vi "Npsv pc test.vi"() -> ()   [LabVIEW 2019]
uses:
  Reverse Polarity.ctl
  Forward Polarity.ctl
  Motion Controller Slot.ctl
  Stepper Output Configuration.ctl
  Axis Select.ctl
  MsgTypeDef.ctl
  DataDef.ctl
  <vilib>/NI/Modbus Library/API/Modbus API.lvclass
  <vilib>/WPC Systems Ltd/GECO Driver/Lib/GECOBase/GECO_Driver Class/GECO_Driver.lvclass
  <vilib>/WPC Systems Ltd/GECO Driver/Lib/GECOMotion/GECOMotion/_typedefine/Axis Select.ctl
  <vilib>/WPC Systems Ltd/GECO Driver/Lib/GECOBase/GECO_Driver Class/Motion/_typedefine/GECO_Stepper Output Configuration.ctl
  <vilib>/WPC Systems Ltd/GECO Driver/Lib/GECOBase/GECO_Driver Class/Motion/_typedefine/GECO_Motion Operation Mode.ctl
  <vilib>/WPC Systems Ltd/GECO Driver/Lib/GECOBase/GECO_Driver Class/GECO_SlotName.ctl
  <vilib>/WPC Systems Ltd/GECO Driver/Lib/GECOBase/GECO_Driver Class/Motion/_typedefine/GECO_ActiveHighLow.ctl
  <vilib>/WPC Systems Ltd/GECO Driver/Lib/GECOMotion/GECOMotion/GECO Motion.lvclass
  GyroDef.ctl
  <vilib>/Instr/_visa.llb/VISA Configure Serial Port (Instr).vi
panel:
  out "RT error out":errorcluster
  out "RT Program Period":u32
  out "error IO 2":errorcluster
  out "error IO":errorcluster
  out "實際角度":cluster{"A":dbl, "B":dbl}={"A"=-3.299667554384925, "B"=3.520332445615068}
  out "實際角度Chart":cluster{"X":dbl, "Y":dbl}(graph)={"X"=-3.299667554384925, "Y"=3.520332445615068} caption="Waveform Chart - dark"
  out "Gyro\nPeriod":u32
  in  "Main Setting Tab":T1(tab)
  in  "TimerON":bool
  in  "Timer(ms)":i32=1
  in  "Serial Port":refnum<visa-resource-name>="COM3"
  in  "TCP slave port":u32=1
  in  "baud rate":u32=115200
  in  "Byte bits":u32=8
  in  "Modbus Address Starting":u32
  in  "Modbus Number of Inputs":u32=10000
  in  "Resource Name":tag="rio://192.168.0.224/RIO0"
  in  "Servo on":bool
  in  "Axis Select":T2
  in  "Stepper Output Configuration":T3=enum."CW/CCW(Two Pulse)"
  in  "Forward Enable?":bool=TRUE
  in  "Reverse Enable?":bool=TRUE
  in  "Motion Operation Mode":T4(ring)=enum."Velocity"
  in  "Forward Polarity":T5
  in  "Reverse Polarity":T6
  in  "Motion Controller Slot":T7
  in  "Target Position (0)":dbl=10000.0
  in  "Acceleration (100000)":u32=300000
  in  "Velocity (10000)":dbl=100000.0
  in  "Deacceleration (100000)":u32=300000
  in  "PID gains setting Tab":enum32{"Axis 1", "Axis 2", "Axis 3"}(tab)
  in  "PID gains":T8={"proportional gain (Kc)"=0.75, "integral time (Ti, min)"=0.01, "derivative time (Td, min)"=0.0} {"derivative time (Td, min)" format="%#_3f"; "integral time (Ti, min)" format="%#_3f"; "proportional gain (Kc)" format="%#_3f"}
  in  "PID gains 2":T8={"proportional gain (Kc)"=0.75, "integral time (Ti, min)"=0.01, "derivative time (Td, min)"=0.0} {"derivative time (Td, min)" format="%#_3f"; "integral time (Ti, min)" format="%#_3f"; "proportional gain (Kc)" format="%#_3f"}
  in  "PID gains 3":T8={"proportional gain (Kc)"=0.75, "integral time (Ti, min)"=0.01, "derivative time (Td, min)"=0.0} {"derivative time (Td, min)" format="%#_3f"; "integral time (Ti, min)" format="%#_3f"; "proportional gain (Kc)" format="%#_3f"}
  in  "ZABStop":bool
  in  "B":i32
  in  "A":i32
  in  "Z":i32=50
  in  "ZAB Start":bool
  in  "Move Setting":T9
  out "Axis 1":T10
  out "Axis 2":T10
  out "Axis 3":T10
  out "Program Period":u32
  in  "ServoButtonControl":T11
  in  "Connect":bool
  in  "Close":bool
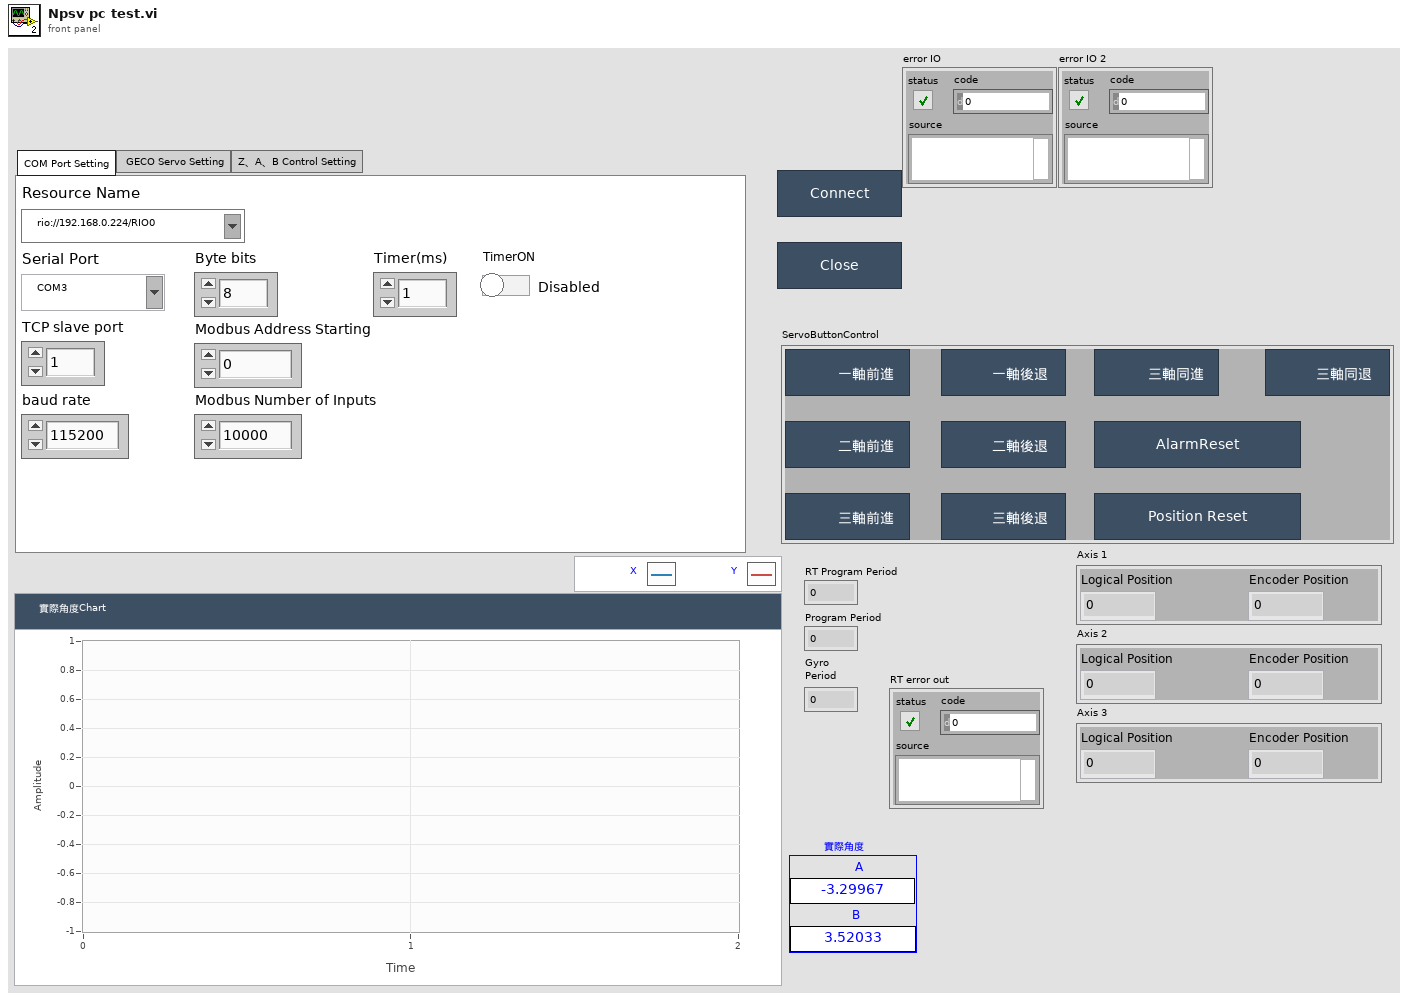
[diagram p1: front panel]
types:
  T1 = enum32{"COM Port Setting", " GECO Servo Setting", "Z、A、B Control Setting"}
  T2 = typedef "Axis Select.ctl" = enum16{"Axis 1", "Axis 2", "Axis 3", "Axis 4"}
  T3 = typedef "Stepper Output Configuration.ctl" = enum16{"Step/Dir(One Pulse)", "CW/CCW(Two Pulse)"}
  T4 = enum16{"Absolute Position", "Relative Position", "Velocity"}
  T5 = typedef "Forward Polarity.ctl" = enum16{"Active High", "Active Low"}
  T6 = typedef "Reverse Polarity.ctl" = enum16{"Active High", "Active Low"}
  T7 = typedef "Motion Controller Slot.ctl" = enum16{"C1", "C2", "C3", "C4"}
  T8 = cluster{"proportional gain (Kc)":dbl, "integral time (Ti, min)":dbl, "derivative time (Td, min)":dbl}
  T9 = typedef "軌跡設定.ctl" = u16
  T10 = cluster{"Encoder Position":i32, "Logical Position":i32}
  T11 = cluster{"三軸同退":bool, "三軸同進":bool, "三軸後退":bool, "三軸前進":bool, "二軸後退":bool, "二軸前進":bool, "一軸後退":bool, "一軸前進":bool, "Reset Encoder Position":bool, "AlarmReset":bool}
  T12 = typedef "GyroDef.ctl" = cluster{"Byte bits":u16, "baud rate":u32, "實際角度":cluster{"A":dbl, "B":dbl}, "COM Port":refnum<visa-resource-name>, "Save Path":refnum<file>}
  T13 = typedef "DataDef.ctl" = cluster{"address starting":u16, "狀態":enum16{"初始化", "讀取", "寫入", "停止"}, "理想角度":cluster{"A":dbl, "B":dbl}, "register values":i16[], "Modbus COM":refnum<class "Modbus API.lvclass">, "TCP slave port":u16, " baud rate":u32, "Byte bits":u16, "ServoButtonControl":cluster{"三軸同退":bool, "三軸同進":bool, "三軸後退":bool, "三軸前進":bool, "二軸後退":bool, "二軸前進":bool, "一軸後退":bool, "一軸前進":bool}, "Serial Number":string, "GECO_Driver out":refnum<class "GECO_Driver.lvclass">, "number of inputs":u16, "ServoSetting":cluster{"Axis Select":T14, "Stepper Output Configuration":T15, "Motion Operation Mode":T16, "Motion Controller Slot":T17, "Singel Axis Move Paramters":cluster{"Motion Operation Mode":T16, "Target Position (0)":i32, "Velocity (10000)":i32, "Acceleration (100000)":u32, "Deacceleration (100000)":u32}, "Reverse":cluster{"Reverse Enable":bool, "Reverse Polarity":T18}, "Forward":cluster{"Forward Enable":bool, "Forward Polarity":T18}}, "GECO Motion out":refnum<class "GECO Motion.lvclass">, "Servo on":bool, "Axis 1 Position":cluster{"Encoder Position":i32, "Logical Position":i32}, "Axis 2 Position":cluster{"Encoder Position":i32, "Logical Position":i32}, "Axis 3 Position":cluster{"Encoder Position":i32, "Logical Position":i32}, "PIDSetting":cluster{"Z":i32, "A":i32, "B":i32, "Move Setting":T19, "Axis Pulse":dbl, "Axis Length":dbl, "PID gains ":cluster{"proportional gain (Kc)":dbl, "integral time (Ti, min)":dbl, "derivative time (Td, min)":dbl}}, "resource name":tag, "Save Path":refnum<file>}
  T14 = typedef "GECO Motion.lvclass/Axis Select.ctl" = enum16{"Axis 1", "Axis 2", "Axis 3", "Axis 4"}
  T15 = typedef "GECO_Driver.lvclass/GECO_Stepper Output Configuration.ctl" = enum16{"Step/Dir(One Pulse)", "CW/CCW(Two Pulse)"}
  T16 = typedef "GECO_Driver.lvclass/GECO_Motion Operation Mode.ctl" = enum16{"Absolute Position", "Relative Position", "Velocity"}
  T17 = typedef "GECO_Driver.lvclass/GECO_SlotName.ctl" = enum16{"C1", "C2", "C3", "C4"}
  T18 = typedef "GECO_Driver.lvclass/GECO_ActiveHighLow.ctl" = enum16{"Active High", "Active Low"}
  T19 = typedef "­y¸ñ.ctl" = u16
  T20 = typedef "MsgTypeDef.ctl" = cluster{"CMD":string, "DATA":variant}
  T21 = enum16{"open", "replace", "create", "open or create", "replace or create", "replace or create with confirmation"}
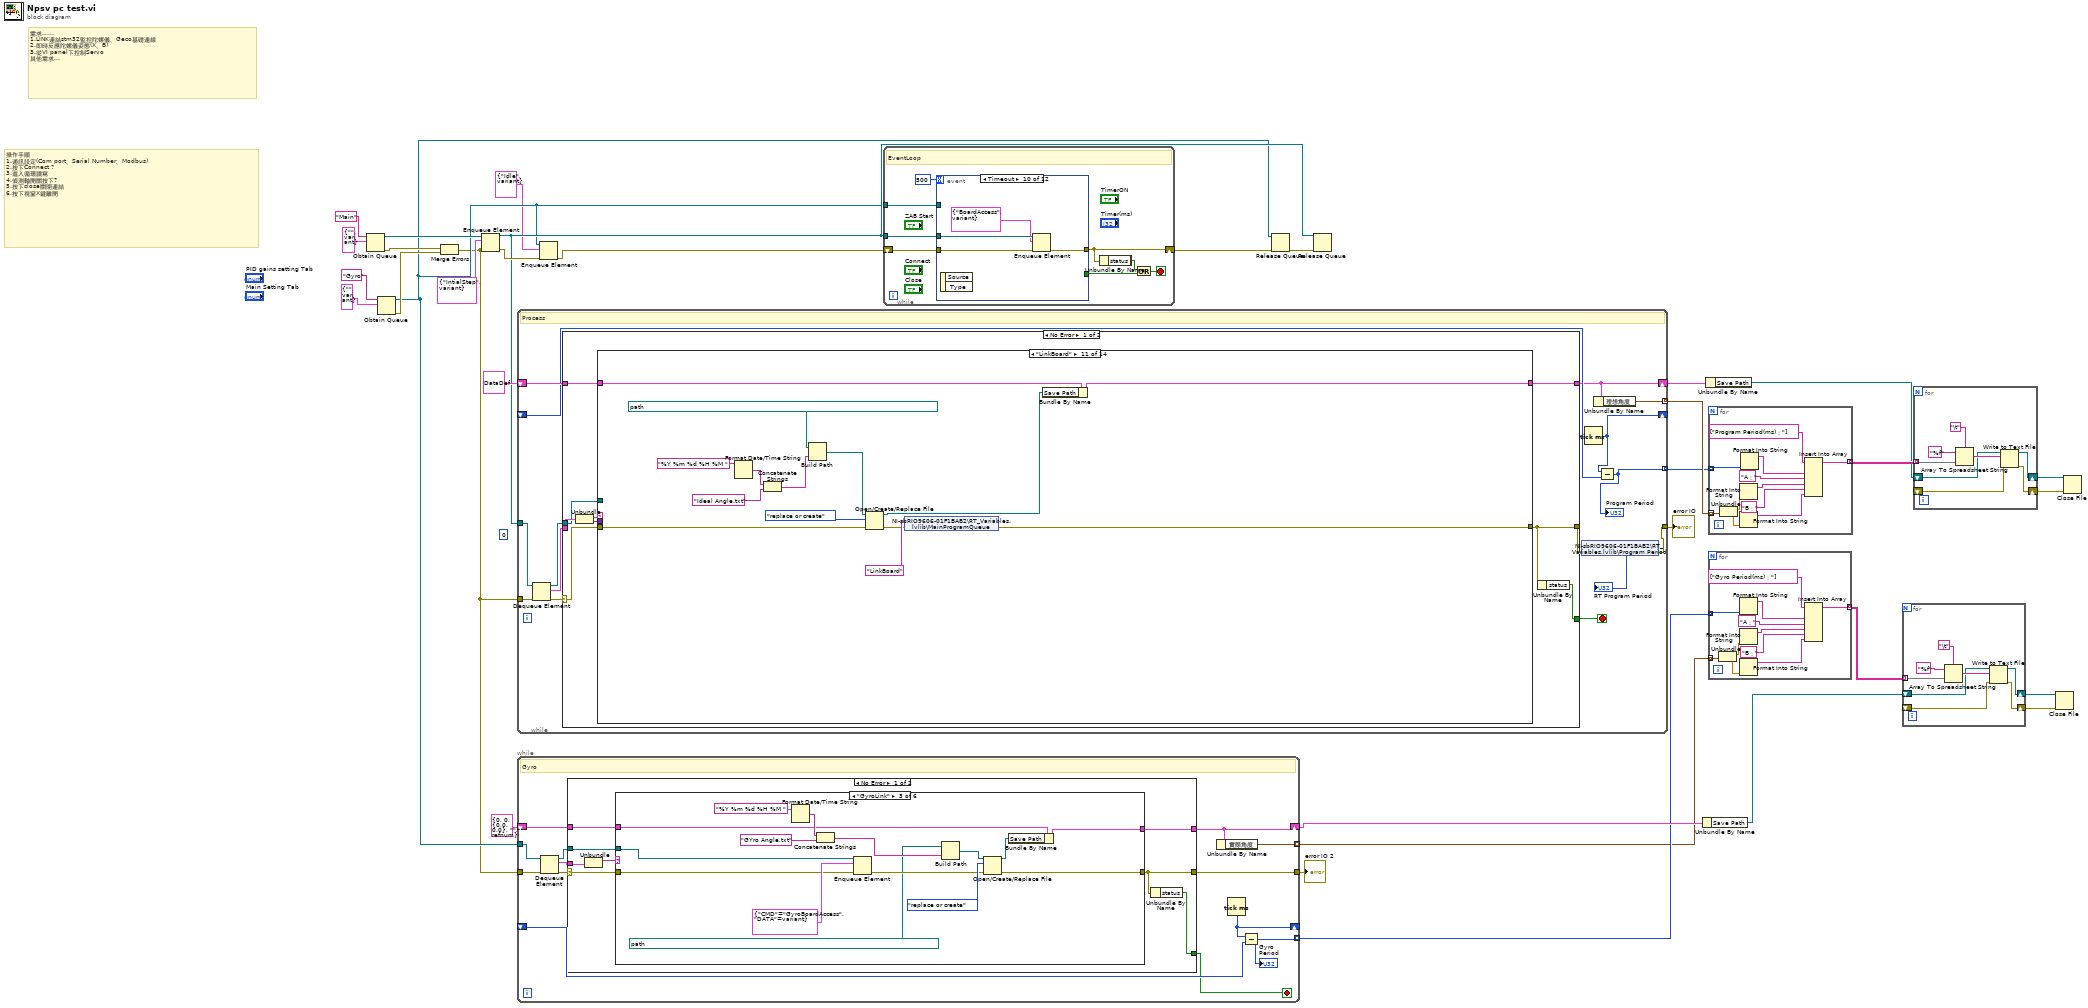
[diagram p0: block diagram]
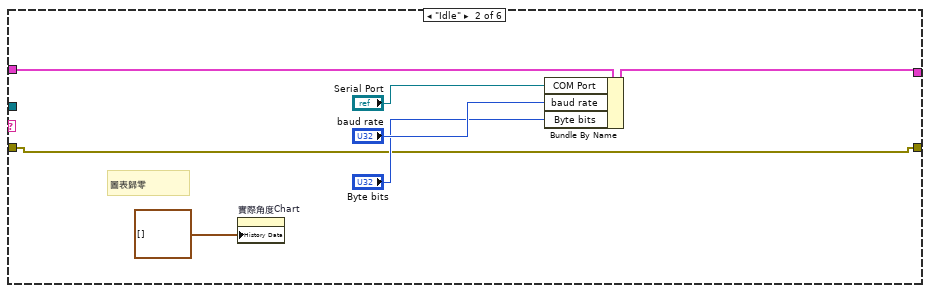
[diagram p3: hidden frame]
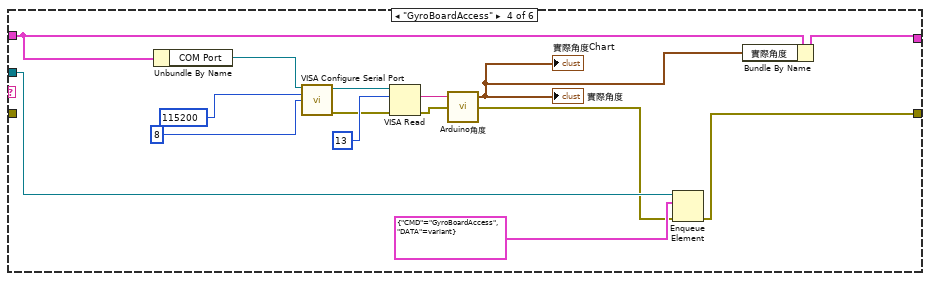
[diagram p4: hidden frame]
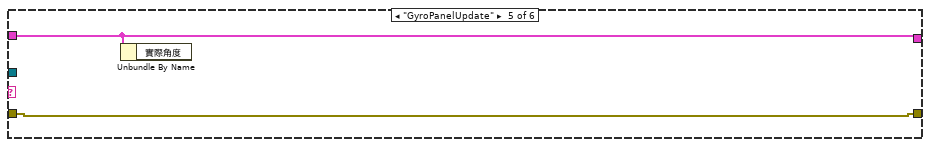
[diagram p5: hidden frame]
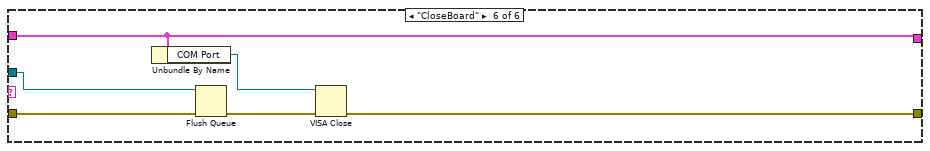
[diagram p6: hidden frame]
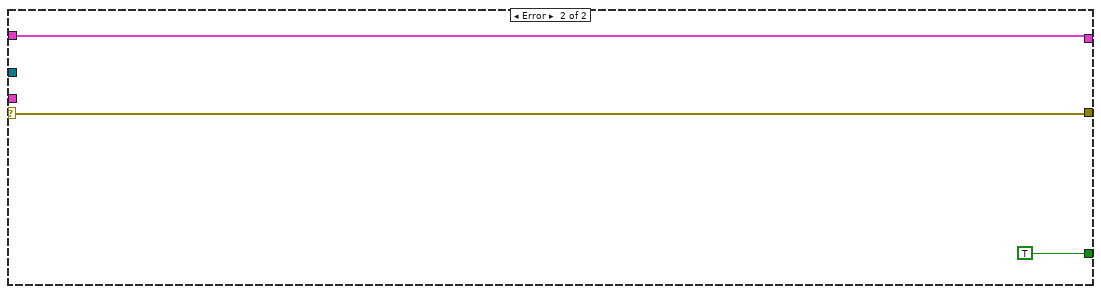
[diagram p7: hidden frame]
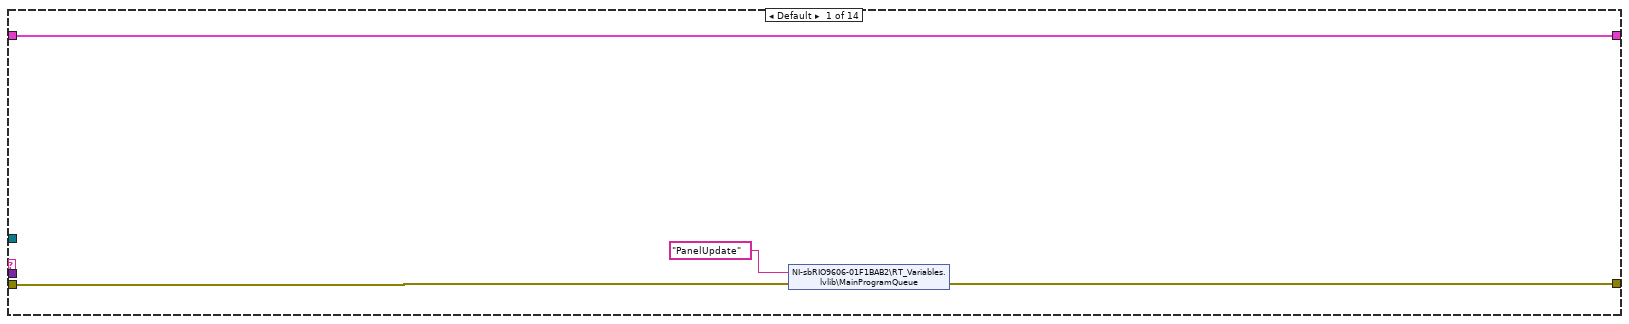
[diagram p8: hidden frame]
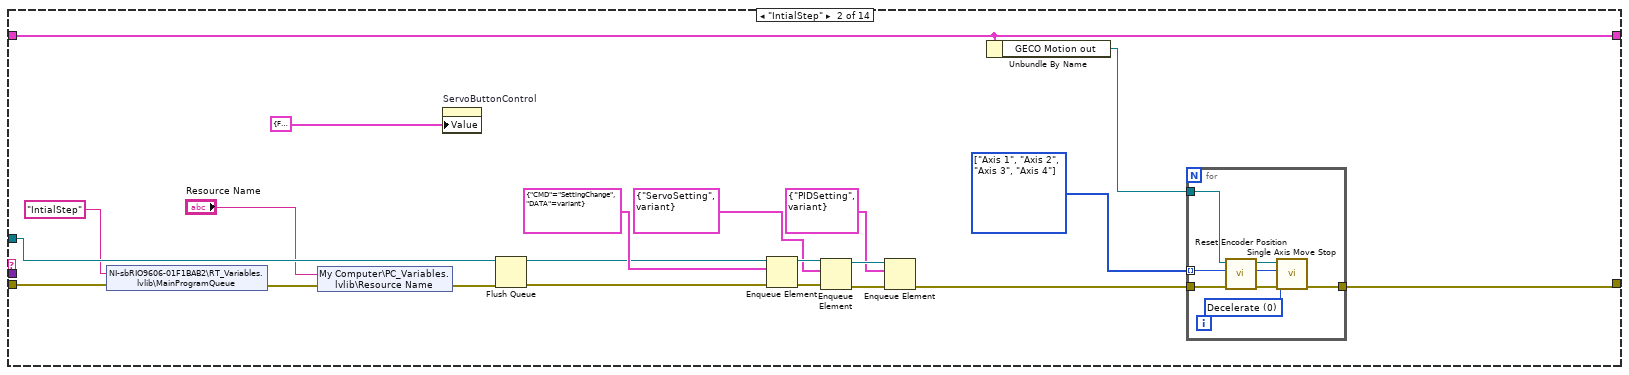
[diagram p9: hidden frame]
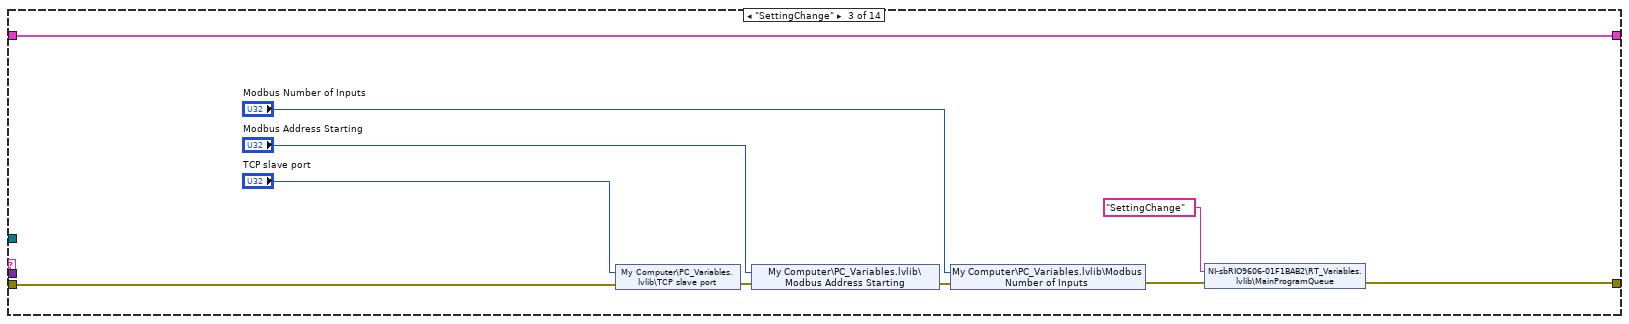
[diagram p10: hidden frame]
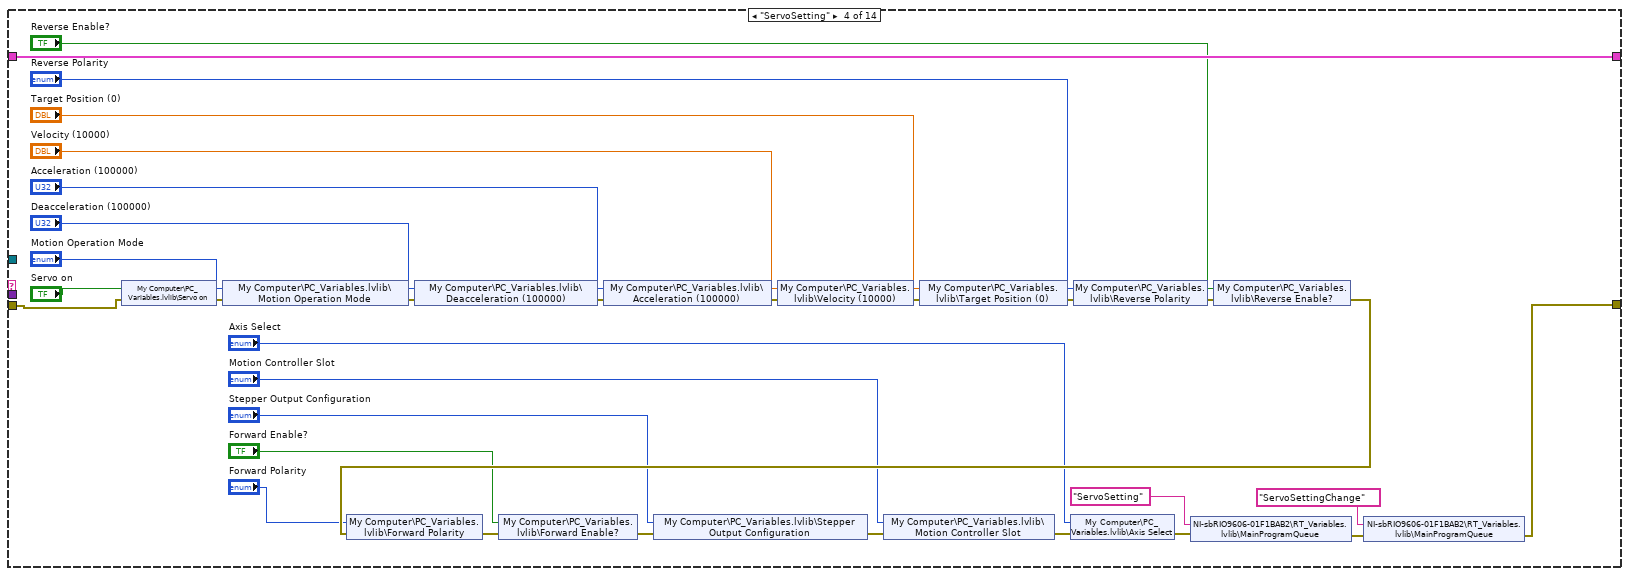
[diagram p11: hidden frame]
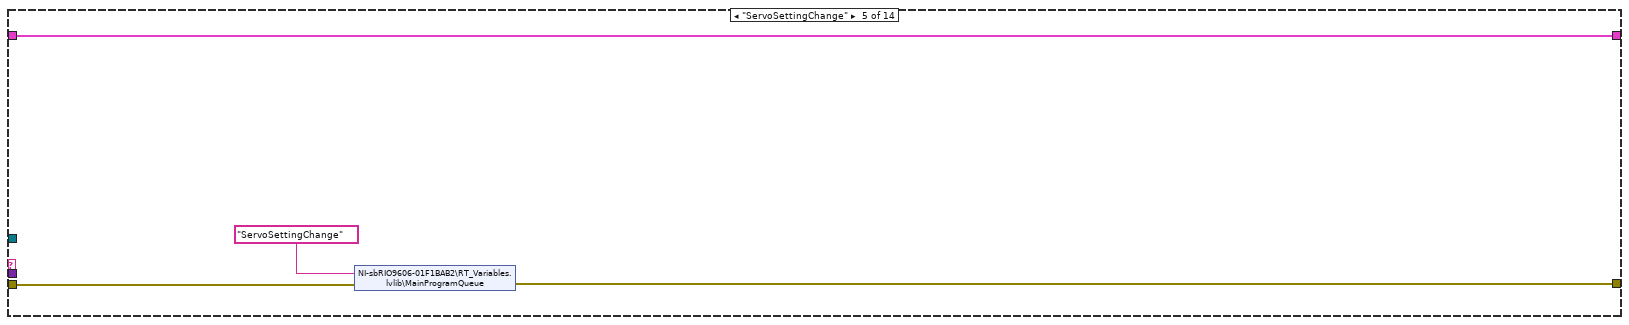
[diagram p12: hidden frame]
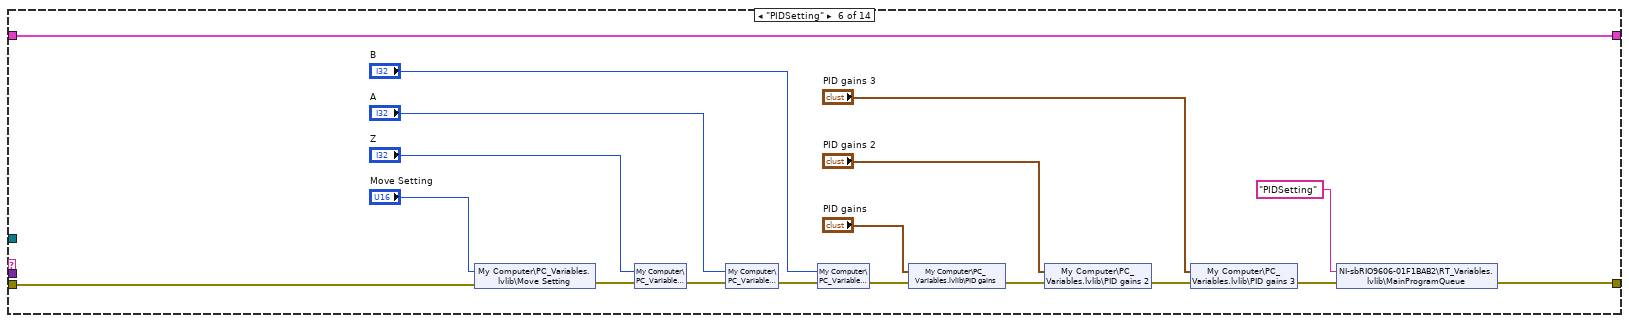
[diagram p13: hidden frame]
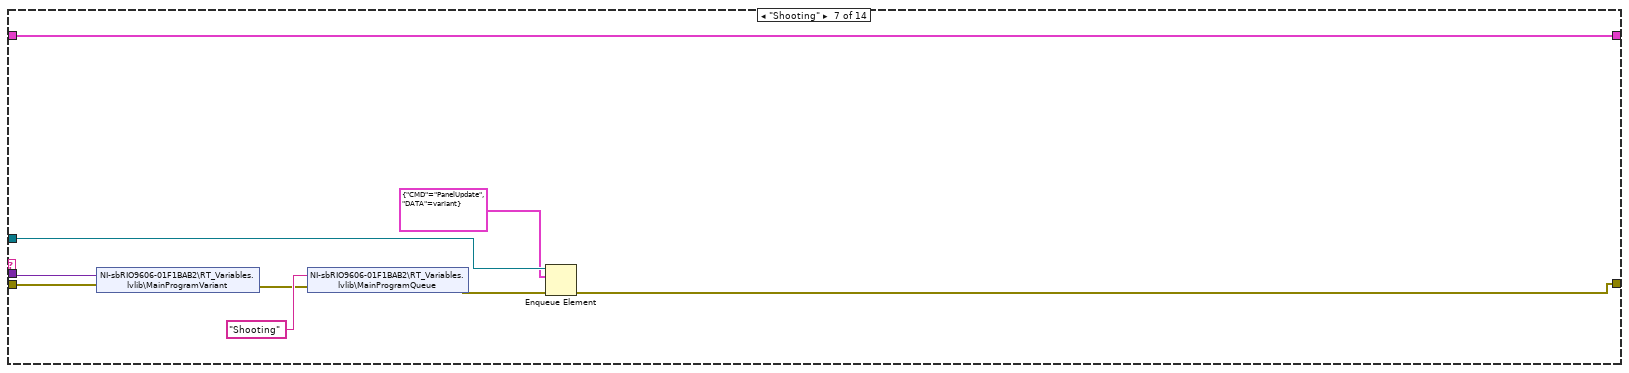
[diagram p14: hidden frame]
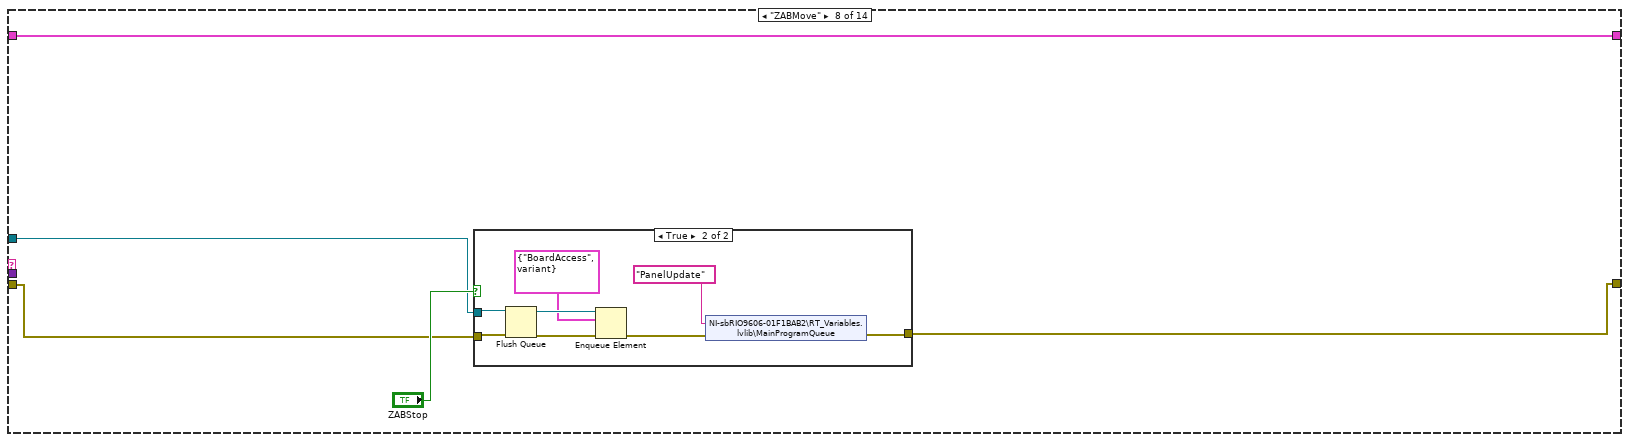
[diagram p15: hidden frame]
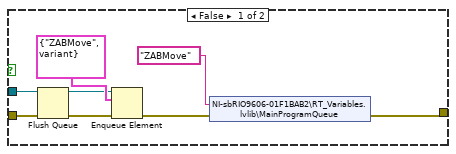
[diagram p16: hidden frame]
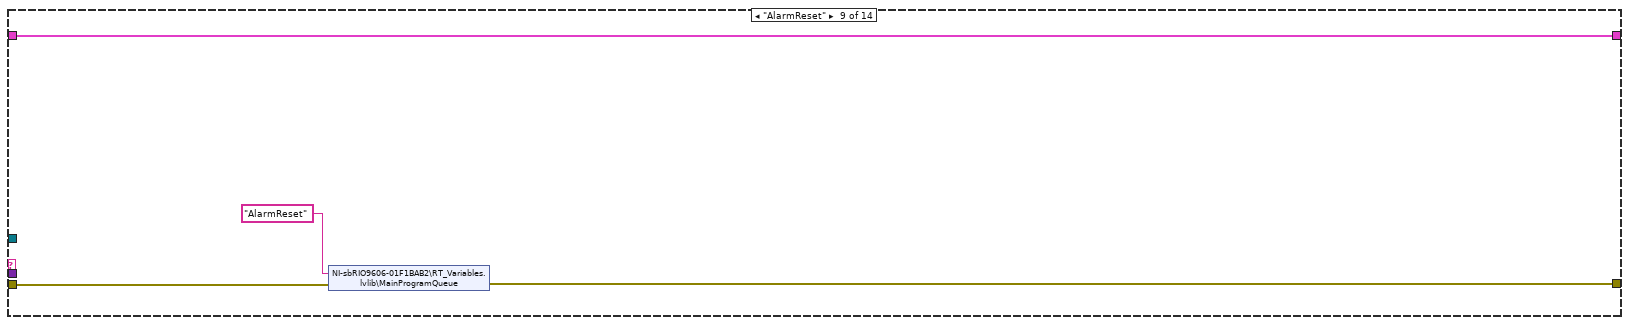
[diagram p17: hidden frame]
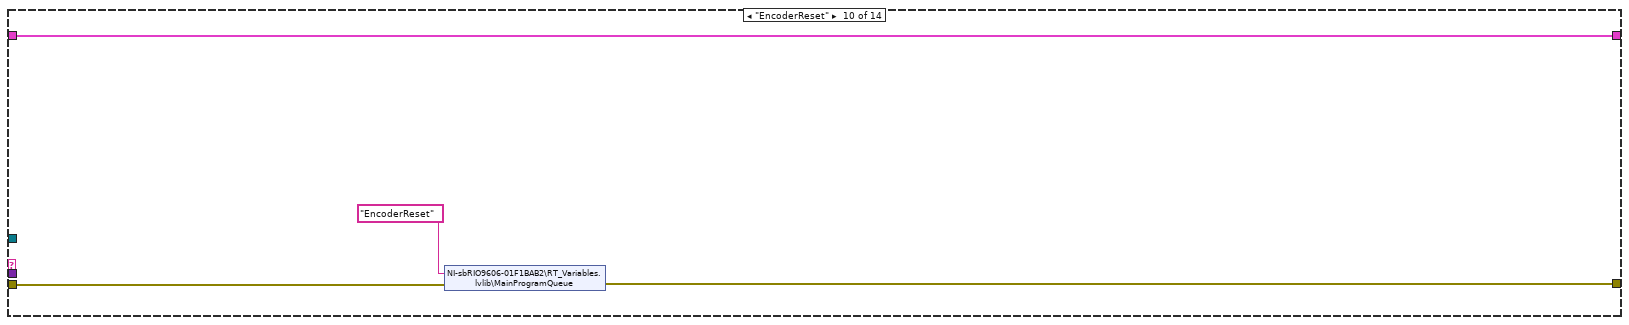
[diagram p18: hidden frame]
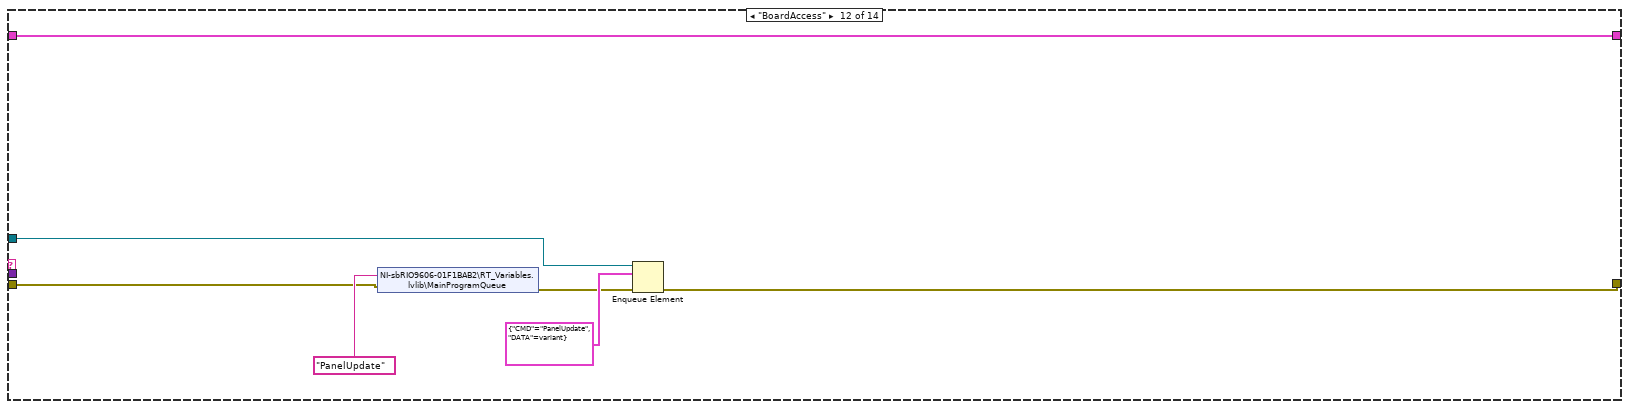
[diagram p19: hidden frame]
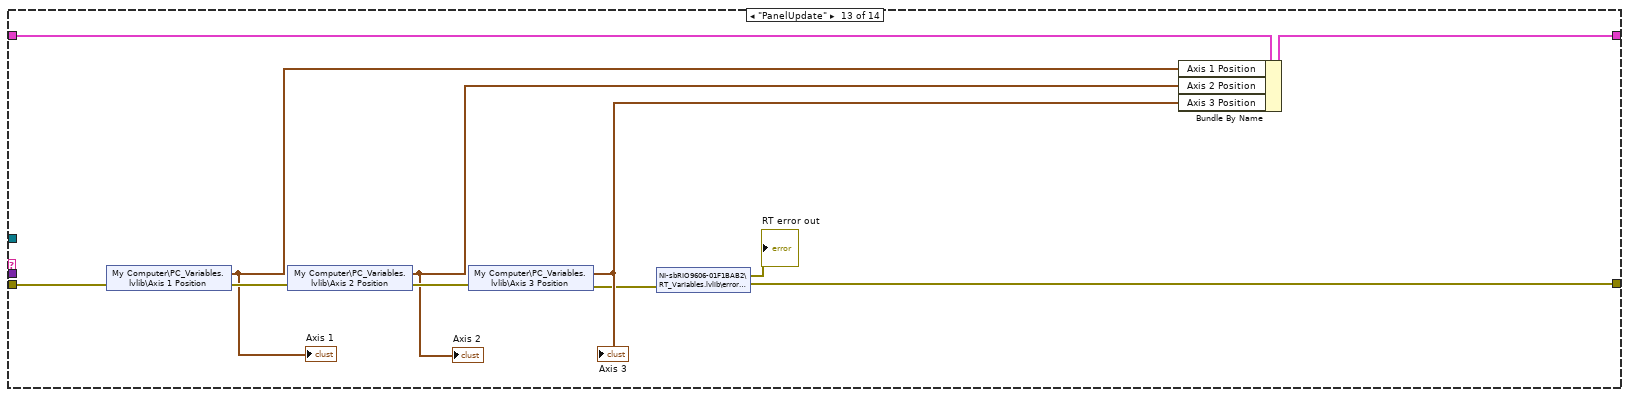
[diagram p20: hidden frame]
diagram:
  (unwired) 0
  # "操作手順\n1.通訊設定(Com port、Serial Number、Modbus)\n2.按下Connect ?\n3.進入循環讀寫\n4.偵測軸開關按下?\n5.按下close關閉連結\n6.按下視窗X鍵離開"
  # "需求......\n1.LINK連結stm32監控陀螺儀、Geco基礎連線\n2.即時反應陀螺儀姿態(X、B)\n3.從VI panel下控制Servo\n其他需求..."
  n1 = Obtain Queue(name (unnamed)="Main", element data type=T20 {"CMD"="", "DATA"=variant}) -> (queue out=w30:refnum<queue>, error out=w25:errorcluster)  [unwired: 3 in, 1 out]
  n2 = Obtain Queue(name (unnamed)="Gyro", element data type=T20 {"CMD"="", "DATA"=variant}) -> (queue out=w20:refnum<queue>, error out=w26:errorcluster)  [unwired: 3 in, 1 out]
  n3 = Merge Errors(w25, w26) -> (w18:errorcluster)
  n4 = Enqueue Element(queue=w30, element=T20 {"CMD"="IntialStep", "DATA"=variant}, error in (no error)=w18) -> (queue out=w21:refnum<queue>, error out=w23:errorcluster)  [unwired: 1 in, 1 out]
  n5 = while {
    tunnel: w21 -> [w49]
    shift-right: [w40] -> w13
    shift-left: T13 {"address starting"=0, "狀態"=enum."初始化", "理想角度"={"A"=0.0, "B"=0.0}, "register values"=[], "Modbus COM"=refnum, "TCP slave port"=1, " baud rate"=0, "Byte bits"=0, "ServoButtonControl"={"三軸同退"=FALSE, "三軸同進"=FALSE, "三軸後退"=FALSE, "三軸前進"=FALSE, "二軸後退"=FALSE, "二軸前進"=FALSE, "一軸後退"=FALSE, "一軸前進"=FALSE}, "Serial Number"="", "GECO_Driver out"=refnum, "number of inputs"=0, "ServoSetting"={"Axis Select"=enum."Axis 1", "Stepper Output Configuration"=enum."Step/Dir(One Pulse)", "Motion Operation Mode"=enum."Absolute Position", "Motion Controller Slot"=enum."C1", "Singel Axis Move Paramters"={"Motion Operation Mode"=enum."Velocity", "Target Position (0)"=10000, "Velocity (10000)"=1, "Acceleration (100000)"=100000, "Deacceleration (100000)"=1}, "Reverse"={"Reverse Enable"=FALSE, "Reverse Polarity"=enum."Active Low"}, "Forward"={"Forward Enable"=FALSE, "Forward Polarity"=enum."Active Low"}}, "GECO Motion out"=refnum, "Servo on"=FALSE, "Axis 1 Position"={"Encoder Position"=0, "Logical Position"=0}, "Axis 2 Position"={"Encoder Position"=0, "Logical Position"=0}, "Axis 3 Position"={"Encoder Position"=0, "Logical Position"=0}, "PIDSetting"={"Z"=10000, "A"=10000, "B"=10000, "Move Setting"=1, "Axis Pulse"=10000.0, "Axis Length"=10000.0, "PID gains "={"proportional gain (Kc)"=1.0, "integral time (Ti, min)"=0.01, "derivative time (Td, min)"=0.0}}, "resource name"="", "Save Path"=refnum} -> [w45]
    tunnel: w18 -> [w43]
    shift-right: [w42] -> _
    shift-left: _ -> [w41]
    tunnel: [w39] -> w16 mode=indexing
    tunnel: [w38] -> w15 mode=indexing
    tunnel: [w36] -> w2
    stop <- w46 stop-if-true
    # "Process"
    n6 = Dequeue Element(queue=w49, error in (no error)=w43) -> (queue out=w44:refnum<queue>, element=w47:T20, error out=w48:errorcluster)  [unwired: 1 in, 1 out]
    n7 = case shown="No Error" w48 {
      selector: w48 -> [w54 w232]
      tunnel: w47 -> [w58 _]
      tunnel: [w51 TRUE] -> w46
      tunnel: [w56 w233] -> w40
      tunnel: w45 -> [w55 w233]
      tunnel: w44 -> [w53 _]
      tunnel: [w50 w232] -> w37
      frame No Error {
        n8 = Unbundle(w58) -> ("CMD"=w57:string, "DATA"=w52:variant)
        n9 = case shown="\"LinkBoard\"" w57 {
          tunnel: [w62 w68 w100 w133 w134 w155 w164 w165 w189 w193 w195 w211 w224 w231] -> w56
          tunnel: w55 -> [w62 w68 w100 w133 w134 w155 w164 w165 w189 w193 w207 w211 w225 w231]
          tunnel: w54 -> [w61 w67 w92 w132 w136 w154 w157 w167 w188 w191 w198 w209 w221 w229]
          tunnel: [w60 w78 w99 w102 w135 w150 w160 w166 w186 w190 w205 w213 w215 w227] -> w50
          tunnel: w53 -> [_ w72 _ _ _ _ w161 w168 _ _ _ w214 _ w230]
          tunnel: w52 -> [_ _ _ _ _ _ w156 _ _ _ _ _ _ _]
          frame Default {
            n10 = shared-variable "NI-sbRIO9606-01F1BAB2\\RT_Variables.lvlib\\MainProgramQueue"("PanelUpdate", error in=w61) -> (error out=w60:errorcluster)
          }
          frame "IntialStep" {
            w76 = T14[] [enum."Axis 1", enum."Axis 2", enum."Axis 3", enum."Axis 4"] items=["Axis 1", "Axis 2", "Axis 3", "Axis 4"]
            n11 = shared-variable "NI-sbRIO9606-01F1BAB2\\RT_Variables.lvlib\\MainProgramQueue"("IntialStep" ("CMD"), error in=w67) -> (error out=w64:errorcluster)
            n12 = shared-variable "My Computer\\PC_Variables.lvlib\\Resource Name"("Resource Name", error in=w64) -> (error out=w63:errorcluster)
            n13 = property on="ServoButtonControl" class="Clust"("Value"=T11 {"三軸同退"=FALSE, "三軸同進"=FALSE, "三軸後退"=FALSE, "三軸前進"=FALSE, "二軸後退"=FALSE, "二軸前進"=FALSE, "一軸後退"=FALSE, "一軸前進"=FALSE, "Reset Encoder Position"=FALSE, "AlarmReset"=FALSE} ("ServoButtonControl")) -> ()  [unwired: 2 in, 2 out]
            n14 = Flush Queue(queue=w72, error in (no error)=w63) -> (queue out=w71:refnum<queue>, error out=w70:errorcluster)  [unwired: 1 out]
            n15 = Enqueue Element(queue=w71, element=T20 {"CMD"="SettingChange", "DATA"=variant}, error in (no error)=w70) -> (queue out=w81:refnum<queue>, error out=w82:errorcluster)  [unwired: 1 in, 1 out]
            n16 = Enqueue Element(queue=w81, element=T20 {"CMD"="ServoSetting", "DATA"=variant}, error in (no error)=w82) -> (queue out=w75:refnum<queue>, error out=w74:errorcluster)  [unwired: 1 in, 1 out]
            n17 = Enqueue Element(queue=w75, element=T20 {"CMD"="PIDSetting", "DATA"=variant}, error in (no error)=w74) -> (error out=w69:errorcluster)  [unwired: 1 in, 2 out]
            n18 = Unbundle By Name(w68) -> ("GECO Motion out"=w77:refnum<class "GECO Motion.lvclass">)
            n19 = for {
              tunnel: w69 -> [w91]
              tunnel: [w85] -> w78
              tunnel: w77 -> [w90]
              tunnel: w76 -> [w89] mode=indexing
              w84 = u16 0 items=["Decelerate", "Halt"] ("Motion Stop Type")
              n20 = call <vilib>:"Reset Encoder Position.vi"("error in (no error)"=w91, "Axis Select"=w89, "GECO Motion in"=w90) -> ("error out"=w88:errorcluster, "Axis Select out"=w87:T14, "GECO Motion out"=w86:refnum<class "GECO Motion.lvclass">)  [unwired: 6 in]
              n21 = call <vilib>:"Single Axis Move Stop.vi"("error in (no error)"=w88, "Motion Stop Type"=w84, "Axis Select"=w87, "GECO Motion in"=w86) -> ("error out"=w85:errorcluster)  [unwired: 5 in, 2 out]
            }
          }
          frame "SettingChange" {
            n22 = shared-variable "My Computer\\PC_Variables.lvlib\\TCP slave port"("TCP slave port", error in=w92) -> (error out=w98:errorcluster)
            n23 = shared-variable "My Computer\\PC_Variables.lvlib\\Modbus Address Starting"("Modbus Address Starting", error in=w98) -> (error out=w97:errorcluster)
            n24 = shared-variable "My Computer\\PC_Variables.lvlib\\Modbus Number of Inputs"("Modbus Number of Inputs", error in=w97) -> (error out=w96:errorcluster)
            n25 = shared-variable "NI-sbRIO9606-01F1BAB2\\RT_Variables.lvlib\\MainProgramQueue"("SettingChange" ("CMD"), error in=w96) -> (error out=w99:errorcluster)
          }
          frame "ServoSetting" {
            n26 = shared-variable "My Computer\\PC_Variables.lvlib\\Servo on"("Servo on", error in=w132) -> (error out=w130:errorcluster)
            n27 = shared-variable "My Computer\\PC_Variables.lvlib\\Motion Operation Mode"("Motion Operation Mode", error in=w130) -> (error out=w129:errorcluster)
            n28 = shared-variable "My Computer\\PC_Variables.lvlib\\Deacceleration (100000)"("Deacceleration (100000)", error in=w129) -> (error out=w128:errorcluster)
            n29 = shared-variable "My Computer\\PC_Variables.lvlib\\Acceleration (100000)"("Acceleration (100000)", error in=w128) -> (error out=w127:errorcluster)
            n30 = shared-variable "My Computer\\PC_Variables.lvlib\\Velocity (10000)"("Velocity (10000)", error in=w127) -> (error out=w126:errorcluster)
            n31 = shared-variable "My Computer\\PC_Variables.lvlib\\Target Position (0)"("Target Position (0)", error in=w126) -> (error out=w125:errorcluster)
            n32 = shared-variable "My Computer\\PC_Variables.lvlib\\Reverse Polarity"("Reverse Polarity", error in=w125) -> (error out=w124:errorcluster)
            n33 = shared-variable "My Computer\\PC_Variables.lvlib\\Reverse Enable?"("Reverse Enable?", error in=w124) -> (error out=w131:errorcluster)
            n34 = shared-variable "My Computer\\PC_Variables.lvlib\\Forward Polarity"("Forward Polarity", error in=w131) -> (error out=w115:errorcluster)
            n35 = shared-variable "My Computer\\PC_Variables.lvlib\\Forward Enable?"("Forward Enable?", error in=w115) -> (error out=w114:errorcluster)
            n36 = shared-variable "My Computer\\PC_Variables.lvlib\\Stepper Output Configuration"("Stepper Output Configuration", error in=w114) -> (error out=w113:errorcluster)
            n37 = shared-variable "My Computer\\PC_Variables.lvlib\\Motion Controller Slot"("Motion Controller Slot", error in=w113) -> (error out=w112:errorcluster)
            n38 = shared-variable "My Computer\\PC_Variables.lvlib\\Axis Select"("Axis Select", error in=w112) -> (error out=w106:errorcluster)
            n39 = shared-variable "NI-sbRIO9606-01F1BAB2\\RT_Variables.lvlib\\MainProgramQueue"("ServoSetting" ("CMD"), error in=w106) -> (error out=w104:errorcluster)
            n40 = shared-variable "NI-sbRIO9606-01F1BAB2\\RT_Variables.lvlib\\MainProgramQueue"("ServoSettingChange" ("CMD"), error in=w104) -> (error out=w102:errorcluster)
          }
          frame "ServoSettingChange" {
            n41 = shared-variable "NI-sbRIO9606-01F1BAB2\\RT_Variables.lvlib\\MainProgramQueue"("ServoSettingChange" ("CMD"), error in=w136) -> (error out=w135:errorcluster)
          }
          frame "PIDSetting" {
            n42 = shared-variable "My Computer\\PC_Variables.lvlib\\Move Setting"("Move Setting", error in=w154) -> (error out=w153:errorcluster)
            n43 = shared-variable "My Computer\\PC_Variables.lvlib\\Z"("Z", error in=w153) -> (error out=w152:errorcluster)
            n44 = shared-variable "My Computer\\PC_Variables.lvlib\\A"("A", error in=w152) -> (error out=w151:errorcluster)
            n45 = shared-variable "My Computer\\PC_Variables.lvlib\\B"("B", error in=w151) -> (error out=w141:errorcluster)
            n46 = shared-variable "My Computer\\PC_Variables.lvlib\\PID gains"("PID gains", error in=w141) -> (error out=w140:errorcluster)
            n47 = shared-variable "My Computer\\PC_Variables.lvlib\\PID gains 2"("PID gains 2", error in=w140) -> (error out=w139:errorcluster)
            n48 = shared-variable "My Computer\\PC_Variables.lvlib\\PID gains 3"("PID gains 3", error in=w139) -> (error out=w138:errorcluster)
            n49 = shared-variable "NI-sbRIO9606-01F1BAB2\\RT_Variables.lvlib\\MainProgramQueue"("PIDSetting", error in=w138) -> (error out=w150:errorcluster)
          }
          frame "Shooting" {
            n50 = shared-variable "NI-sbRIO9606-01F1BAB2\\RT_Variables.lvlib\\MainProgramVariant"(w156, error in=w157) -> (error out=w158:errorcluster)
            n51 = shared-variable "NI-sbRIO9606-01F1BAB2\\RT_Variables.lvlib\\MainProgramQueue"("Shooting" ("CMD"), error in=w158) -> (error out=w162:errorcluster)
            n52 = Enqueue Element(queue=w161, element=T20 {"CMD"="PanelUpdate", "DATA"=variant}, error in (no error)=w162) -> (error out=w160:errorcluster)  [unwired: 1 in, 2 out]
          }
          frame "ZABMove" {
            n53 = case shown="True" "ZABStop" {
              tunnel: [w171 w179] -> w166
              tunnel: w168 -> [w174 w182]
              tunnel: w167 -> [w173 w181]
              frame False {
                n54 = Flush Queue(queue=w174, error in (no error)=w173) -> (queue out=w175:refnum<queue>, error out=w176:errorcluster)  [unwired: 1 out]
                n55 = Enqueue Element(queue=w175, element=T20 {"CMD"="ZABMove", "DATA"=variant}, error in (no error)=w176) -> (error out=w172:errorcluster)  [unwired: 1 in, 2 out]
                n56 = shared-variable "NI-sbRIO9606-01F1BAB2\\RT_Variables.lvlib\\MainProgramQueue"("ZABMove" ("CMD"), error in=w172) -> (error out=w171:errorcluster)
              }
              frame True {
                n57 = Flush Queue(queue=w182, error in (no error)=w181) -> (queue out=w185:refnum<queue>, error out=w184:errorcluster)  [unwired: 1 out]
                n58 = Enqueue Element(queue=w185, element=T20 {"CMD"="BoardAccess", "DATA"=variant}, error in (no error)=w184) -> (error out=w178:errorcluster)  [unwired: 1 in, 2 out]
                n59 = shared-variable "NI-sbRIO9606-01F1BAB2\\RT_Variables.lvlib\\MainProgramQueue"("PanelUpdate" ("CMD"), error in=w178) -> (error out=w179:errorcluster)
              }
            }
          }
          frame "AlarmReset" {
            n60 = shared-variable "NI-sbRIO9606-01F1BAB2\\RT_Variables.lvlib\\MainProgramQueue"("AlarmReset", error in=w188) -> (error out=w186:errorcluster)
          }
          frame "EncoderReset" {
            n61 = shared-variable "NI-sbRIO9606-01F1BAB2\\RT_Variables.lvlib\\MainProgramQueue"("EncoderReset", error in=w191) -> (error out=w190:errorcluster)
          }
          frame "LinkBoard" {
            n62 = Format Date/Time String(time format string (%c)="%Y %m %d %H %M ") -> (date/time string=w203:string)  [unwired: 2 in]
            n63 = Concatenate Strings(w203, "Ideal Angle.txt" ("element")) -> (w202:string)
            n64 = Build Path(base path=path "C:/Users/user/Desktop/軸卡/labview/碩論/陀螺儀監控平台控制/SbRioControl/SbRIoGyroData", name or relative path=w202) -> (appended path=w196:path)
            n65 = Open/Create/Replace File(file path (use dialog)=w196, error in=w198, operation (0:open)=T21."replace or create") -> (refnum out=w194:refnum<file>, error out=w199:errorcluster)  [unwired: 3 in, 1 out]
            n66 = shared-variable "NI-sbRIO9606-01F1BAB2\\RT_Variables.lvlib\\MainProgramQueue"("LinkBoard", error in=w199) -> (error out=w205:errorcluster)
            n67 = Bundle By Name(cluster=w207, "Save Path"=w194) -> (w195:T13)
          }
          frame "BoardAccess" {
            n68 = shared-variable "NI-sbRIO9606-01F1BAB2\\RT_Variables.lvlib\\MainProgramQueue"("PanelUpdate", error in=w209) -> (error out=w208:errorcluster)
            n69 = Enqueue Element(queue=w214, element=T20 {"CMD"="PanelUpdate", "DATA"=variant}, error in (no error)=w208) -> (error out=w213:errorcluster)  [unwired: 1 in, 2 out]
          }
          frame "PanelUpdate" {
            n70 = shared-variable "My Computer\\PC_Variables.lvlib\\Axis 1 Position"(error in=w221) -> (w220:T10, error out=w223:errorcluster)
            "Axis 1" <- w220
            n71 = shared-variable "My Computer\\PC_Variables.lvlib\\Axis 2 Position"(error in=w223) -> (w219:T10, error out=w222:errorcluster)
            "Axis 2" <- w219
            n72 = shared-variable "My Computer\\PC_Variables.lvlib\\Axis 3 Position"(error in=w222) -> (w218:T10, error out=w216:errorcluster)
            "Axis 3" <- w218
            n73 = shared-variable "NI-sbRIO9606-01F1BAB2\\RT_Variables.lvlib\\error out"(error in=w216) -> (→"RT error out":errorcluster, error out=w215:errorcluster)
            n74 = Bundle By Name(cluster=w225, "Axis 1 Position"=w220, "Axis 2 Position"=w219, "Axis 3 Position"=w218) -> (w224:T13)
          }
          frame "CloseBoard" {
            n75 = Flush Queue(queue=w230, error in (no error)=w229) -> (error out=w228:errorcluster)  [unwired: 2 out]
            n76 = shared-variable "NI-sbRIO9606-01F1BAB2\\RT_Variables.lvlib\\MainProgramQueue"("CloseBoard", error in=w228) -> (error out=w227:errorcluster)
          }
        }
        n77 = Unbundle By Name(w50) -> ("status"=w51:bool)
      }
      frame Error {
      }
    }
    n78 = shared-variable "NI-sbRIO9606-01F1BAB2\\RT_Variables.lvlib\\Program Period"(error in=w37) -> (→"RT Program Period":u32, error out=w36:errorcluster)
    n79 = Tick Count (ms)() -> (millisecond timer value=w42:u32)
    n80 = Unbundle By Name(w40) -> ("理想角度"=w39:cluster{"A":dbl, "B":dbl})
    n81 = Subtract(x=w42, y=w41) -> (x-y=w38:u32)
    "Program Period" <- w38
  }
  "error IO" <- w2
  n82 = while {
    tunnel: w20 -> [w247]
    tunnel: w18 -> [w246]
    shift-right: [w241] -> w11
    shift-left: T12 {"Byte bits"=0, "baud rate"=0, "實際角度"={"A"=0.0, "B"=0.0}, "COM Port"="", "Save Path"=refnum} -> [w242]
    tunnel: [w240] -> w4 mode=indexing
    shift-right: [w239] -> _
    shift-left: _ -> [w238]
    tunnel: [w236] -> w1
    tunnel: [w235] -> w5 mode=indexing
    stop <- w237 stop-if-true
    # "Gyro"
    n83 = Dequeue Element(queue=w247, error in (no error)=w246) -> (queue out=w244:refnum<queue>, element=w243:T20, error out=w245:errorcluster)  [unwired: 1 in, 1 out]
    n84 = case shown="No Error" w245 {
      selector: w245 -> [w251 w303]
      tunnel: w244 -> [w250 _]
      tunnel: w243 -> [w255 _]
      tunnel: [w249 TRUE] -> w237
      tunnel: w242 -> [w253 w304]
      tunnel: [w252 w304] -> w241
      tunnel: [w248 w303] -> w236
      frame No Error {
        n85 = Unbundle(w255) -> ("CMD"=w254:string)  [unwired: 1 out]
        n86 = case shown="\"GyroLink\"" w254 {
          tunnel: [w257 w263 w268 w281 w296 w298] -> w252
          tunnel: w253 -> [w257 w264 w265 w291 w296 w298]
          tunnel: w251 -> [w256 w259 w271 _ w295 w302]
          tunnel: [w256 w259 w269 w287 w295 w299] -> w248
          tunnel: w250 -> [_ _ w278 w290 _ w300]
          frame Default {
          }
          frame "Idle" {
            # "圖表歸零"
            n87 = property on="實際角度Chart" class="WFChart (strict)"("History Data"=cluster{"X":dbl, "Y":dbl}[] []) -> ()  [unwired: 2 in, 2 out]
            n88 = Bundle By Name(cluster=w264, "COM Port"="Serial Port", "baud rate"="baud rate", "Byte bits"="Byte bits") -> (w263:T12)
          }
          frame "GyroLink" {
            n89 = Format Date/Time String(time format string (%c)="%Y %m %d %H %M ") -> (date/time string=w276:string)  [unwired: 2 in]
            n90 = Concatenate Strings(w276, "GYro Angle.txt" ("element")) -> (w273:string)
            n91 = Enqueue Element(queue=w278, element=T20 {"CMD"="GyroBoardAccess", "DATA"=variant}, error in (no error)=w271) -> (error out=w270:errorcluster)  [unwired: 1 in, 2 out]
            n92 = Build Path(base path=path "C:/Users/user/Desktop/軸卡/labview/碩論/陀螺儀監控平台控制/SbRioControl/SbRIoGyroData", name or relative path=w273) -> (appended path=w272:path)
            n93 = Open/Create/Replace File(file path (use dialog)=w272, error in=w270, operation (0:open)=T21."replace or create") -> (refnum out=w267:refnum<file>, error out=w269:errorcluster)  [unwired: 3 in, 1 out]
            n94 = Bundle By Name(cluster=w265, "Save Path"=w267) -> (w268:T12)
          }
          frame "GyroBoardAccess" {
            n95 = Unbundle By Name(w291) -> ("COM Port"=w284:refnum<visa-resource-name>)
            n96 = call-poly "VISA Configure Serial Port"("VISA resource name"=w284, "baud rate (9600)"=u32 115200, "data bits (8)"=u16 8) -> ("VISA resource name out"=w283:refnum<visa-resource-name>, "error out"=w282:errorcluster)  [unwired: 11 in]
            n97 = VISA Read(VISA resource name=w283, byte count=u32 13, error in (no error)=w282) -> (read buffer=w294:string, error out=w293:errorcluster)  [unwired: 2 out]
            n98 = call "Arduino角度.vi"("error in"=w293, "read buffer"=w294) -> ("error out"=w288:errorcluster, "Waveform Chart"=w280:cluster{dbl, dbl})  [unwired: 2 in]
            "實際角度" <- w280
            "實際角度Chart" <- w280
            n99 = Enqueue Element(queue=w290, element=T20 {"CMD"="GyroBoardAccess", "DATA"=variant}, error in (no error)=w288) -> (error out=w287:errorcluster)  [unwired: 1 in, 2 out]
            n100 = Bundle By Name(cluster=w291, "實際角度"=w280) -> (w281:T12)
          }
          frame "GyroPanelUpdate" {
            n101 = Unbundle By Name(w296) -> ()  [unwired: 1 out]
          }
          frame "CloseBoard" {
            n102 = Unbundle By Name(w298) -> ("COM Port"=w297:refnum<visa-resource-name>)
            n103 = Flush Queue(queue=w300, error in (no error)=w302) -> (error out=w301:errorcluster)  [unwired: 2 out]
            n104 = VISA Close(VISA resource name=w297, error in (no error)=w301) -> (error out=w299:errorcluster)
          }
        }
        n105 = Unbundle By Name(w248) -> ("status"=w249:bool)
      }
      frame Error {
      }
    }
    n106 = Unbundle By Name(w241) -> ("實際角度"=w240:cluster{"A":dbl, "B":dbl})
    n107 = Tick Count (ms)() -> (millisecond timer value=w239:u32)
    n108 = Subtract(x=w239, y=w238) -> (x-y=w235:u32)
    "Gyro\nPeriod" <- w235
  }
  "error IO 2" <- w1
  n109 = Enqueue Element(queue=w20, element=T20 {"CMD"="Idle", "DATA"=variant}, error in (no error)=w23) -> (error out=w22:errorcluster)  [unwired: 1 in, 2 out]
  n110 = while {
    shift-right: [w309] -> w34
    shift-left: w22 -> [w312]
    tunnel: w21 -> [w313]
    tunnel: w20 -> [w307]
    stop <- w310 stop-if-true
    # "EventLoop"
    n111 = event shown="[9] Timeout" {
      selector: _ -> [_ _ _ _ _ _ _ _ _ _ _ _]
      dyn-events: _ -> [_ _ _ _ _ _ _ _ _ _ _ _]
      timeout: 500 -> [_ _ _ _ _ _ _ _ _ _ _ _]
      tunnel: w313 -> [w317 w321 w325 w332 w336 w340 w346 w350 _ w358 w366 w369]
      tunnel: w312 -> [w316 w320 w324 w331 w335 w339 w345 w349 w356 w360 w365 w371]
      tunnel: [w315 w319 w323 w328 w334 w338 w344 w348 w355 w359 w363 w368] -> w309
      tunnel: [_ _ _ _ _ _ _ _ _ _ _ w373] -> w311
      tunnel: w307 -> [_ _ _ w326 _ _ _ _ w353 _ w361 w372]
      event "Modbus Number of Inputs", "Serial Port", "TCP slave port", "baud rate", "Byte bits", "Modbus Address Starting": Value Change {
        n112 = event-data() -> ()  [unwired: 1 in, 1 out]
        n113 = Enqueue Element(queue=w317, element=T20 {"CMD"="SettingChange", "DATA"=variant}, error in (no error)=w316) -> (error out=w315:errorcluster)  [unwired: 1 in, 2 out]
      }
      event "Forward Enable?", "Reverse Enable?", "Motion Operation Mode", "Target Position (0)", "Acceleration (100000)", "Velocity (10000)", "Deacceleration (100000)", "Servo on": Value Change {
        n114 = event-data() -> ()  [unwired: 1 in, 1 out]
        n115 = Enqueue Element(queue=w321, element=T20 {"CMD"="ServoSetting", "DATA"=variant}, error in (no error)=w320) -> (error out=w319:errorcluster)  [unwired: 1 in, 2 out]
      }
      event "Z", "A", "B": Value Change {
        n116 = event-data() -> ()  [unwired: 1 in, 2 out]
        n117 = Enqueue Element(queue=w325, element=T20 {"CMD"="PIDSetting", "DATA"=variant}, error in (no error)=w324) -> (error out=w323:errorcluster)  [unwired: 1 in, 2 out]
      }
      event "Connect": Value Change {
        n118 = event-data() -> ()  [unwired: 1 in, 1 out]
        n119 = Enqueue Element(queue=w332, element=T20 {"CMD"="LinkBoard", "DATA"=variant}, error in (no error)=w331) -> (error out=w329:errorcluster)  [unwired: 1 in, 2 out]
        n120 = Enqueue Element(queue=w326, element=T20 {"CMD"="GyroLink", "DATA"=variant}, error in (no error)=w329) -> (error out=w328:errorcluster)  [unwired: 1 in, 2 out]
      }
      event "ServoButtonControl.AlarmReset": Value Change {
        n121 = event-data() -> ()  [unwired: 1 in, 1 out]
        n122 = Enqueue Element(queue=w336, element=T20 {"CMD"="AlarmReset", "DATA"=variant}, error in (no error)=w335) -> (error out=w334:errorcluster)  [unwired: 1 in, 2 out]
      }
      event "ServoButtonControl.Reset Encoder Position": Value Change {
        n123 = event-data() -> ()  [unwired: 1 in, 1 out]
        n124 = Enqueue Element(queue=w340, element=T20 {"CMD"="EncoderReset", "DATA"=variant}, error in (no error)=w339) -> (error out=w338:errorcluster)  [unwired: 1 in, 2 out]
      }
      event "ServoButtonControl": Value Change {
        n125 = event-data() -> ()  [unwired: 1 in, 1 out]
        n126 = Bundle By Name(cluster=T20 {"CMD"="Shooting", "DATA"=variant} ("element"), "DATA"="ServoButtonControl") -> (w342:T20)
        n127 = Enqueue Element(queue=w346, element=w342, error in (no error)=w345) -> (error out=w344:errorcluster)  [unwired: 1 in, 2 out]
      }
      event "ZABStop", "ZAB Start": Value Change {
        n128 = event-data() -> ()  [unwired: 1 in, 2 out]
        n129 = Enqueue Element(queue=w350, element=T20 {"CMD"="ZABMove", "DATA"=variant}, error in (no error)=w349) -> (error out=w348:errorcluster)  [unwired: 1 in, 2 out]
      }
      event "TimerON": Value Change {
        n130 = event-data() -> ("NewVal"=w351:bool)  [unwired: 1 in]
        n131 = Bundle By Name(cluster=T20 {"CMD"="ChangeTimerState", "DATA"=variant} ("element"), "DATA"=w351) -> (w352:T20)
        n132 = Enqueue Element(queue=w353, element=w352, error in (no error)=w356) -> (error out=w355:errorcluster)  [unwired: 1 in, 2 out]
      }
      event Timeout {
        n133 = event-data() -> ()  [unwired: 1 in, 2 out]
        n134 = Enqueue Element(queue=w358, element=T20 {"CMD"="BoardAccess", "DATA"=variant}, error in (no error)=w360) -> (error out=w359:errorcluster)  [unwired: 1 in, 2 out]
      }
      event "Close": Value Change {
        w362 = T20 {"CMD"="CloseBoard", "DATA"=variant} ("element")
        n135 = event-data() -> ()  [unwired: 1 in, 1 out]
        n136 = Enqueue Element At Opposite End(queue=w366, element=w362, error in (no error)=w365) -> (error out=w364:errorcluster)  [unwired: 1 in, 2 out]
        n137 = Enqueue Element At Opposite End(queue=w361, element=w362, error in (no error)=w364) -> (error out=w363:errorcluster)  [unwired: 1 in, 2 out]
      }
      event Panel Close? {
        w367 = T20 {"CMD"="CloseBoard", "DATA"=variant} ("element")
        w373 = TRUE
        n138 = event-data() -> ()  [unwired: 1 in, 1 out]
        n139 = Enqueue Element At Opposite End(queue=w372, element=w367, error in (no error)=w371) -> (error out=w370:errorcluster)  [unwired: 1 in, 2 out]
        n140 = event-data("Discard?"=w373) -> ()  [unwired: 1 in, 1 out]
        n141 = Enqueue Element At Opposite End(queue=w369, element=w367, error in (no error)=w370) -> (error out=w368:errorcluster)  [unwired: 1 in, 2 out]
      }
    }
    n142 = Unbundle By Name(w309) -> ("status"=w308:bool)
    n143 = Or(x=w308, y=w311) -> (x .or. y?=w310:bool)
  }
  n144 = Release Queue(queue=w20, error in (no error)=w34) -> (error out=w24:errorcluster)  [unwired: 1 in, 2 out]
  n145 = Release Queue(queue=w21, error in (no error)=w24) -> ()  [unwired: 1 in, 3 out]
  n146 = Unbundle By Name(w11) -> ("Save Path"=w10:refnum<file>)
  n147 = Unbundle By Name(w13) -> ("Save Path"=w12:refnum<file>)
  n148 = for {
    tunnel: [w383] -> w3 mode=indexing
    tunnel: w4 -> [w382] mode=indexing
    tunnel: w5 -> [w379] mode=indexing
    n149 = Unbundle(w382) -> ("A"=w381:dbl, "B"=w380:dbl)
    n150 = Format Into String(w381) -> (resulting string=w376:string)  [unwired: 3 in, 1 out]
    n151 = Format Into String(w380) -> (resulting string=w375:string)  [unwired: 3 in, 1 out]
    n152 = Format Into String(w379) -> (resulting string=w378:string)  [unwired: 3 in, 1 out]
    n153 = Insert Into Array(array=string[] ["Gyro Period(ms)："], new element #1=w378, new element #2="A：", new element #3=w376, new element #4="B：", new element #5=w375) -> (w383:string[])  [unwired: 1 in]
  }
  n154 = for {
    tunnel: [w394] -> w14 mode=indexing
    tunnel: w16 -> [w393] mode=indexing
    tunnel: w15 -> [w390] mode=indexing
    n155 = Unbundle(w393) -> ("A"=w392:dbl, "B"=w391:dbl)
    n156 = Format Into String(w392) -> (resulting string=w387:string)  [unwired: 3 in, 1 out]
    n157 = Format Into String(w391) -> (resulting string=w385:string)  [unwired: 3 in, 1 out]
    n158 = Format Into String(w390) -> (resulting string=w389:string)  [unwired: 3 in, 1 out]
    n159 = Insert Into Array(array=string[] ["Program Period(ms)："], new element #1=w389, new element #2="A：", new element #3=w387, new element #4="B：", new element #5=w385) -> (w394:string[])  [unwired: 1 in]
  }
  n160 = for {
    shift-right: [w398] -> w8
    shift-left: w10 -> [w400]
    shift-right: [w399] -> w9
    shift-left: _ -> [w397]
    tunnel: w3 -> [w396] mode=indexing
    n161 = Array To Spreadsheet String(delimiter (Tab)="\t", array=w396, 3:"%f" ("format string")) -> (spreadsheet string=w401:string)
    n162 = Write to Text File(file (use dialog)=w400, text=w401, error in=w397) -> (refnum out=w398:refnum<file>, error out=w399:errorcluster)  [unwired: 1 in, 1 out]
  }
  n163 = for {
    tunnel: w14 -> [w406] mode=indexing
    shift-right: [w404] -> w6
    shift-left: w12 -> [w408]
    shift-right: [w405] -> w7
    shift-left: _ -> [w407]
    n164 = Array To Spreadsheet String(delimiter (Tab)="\t", array=w406, 3:"%f" ("format string")) -> (spreadsheet string=w409:string)
    n165 = Write to Text File(file (use dialog)=w408, text=w409, error in=w407) -> (refnum out=w404:refnum<file>, error out=w405:errorcluster)  [unwired: 1 in, 1 out]
  }
  n166 = Close File(refnum=w8, error in=w9) -> ()  [unwired: 2 out]
  n167 = Close File(refnum=w6, error in=w7) -> ()  [unwired: 2 out]
